vi "FRIC_navX_Get_Quaternion.vi"(6 "Zero":bool, 7 "Update":bool) -> (2 "Quaternion":T1)   [LabVIEW 2015, in "navX AE v1.lvlib"]
doc: "This navX VI returns the quaternion of the navX."
uses:
  navX AE v1.lvlib
  navX Library v2/_TypeDefs/Z900_navX_DeviceRegisters.ctl
  navX Library v2/navX Library v2.lvlib
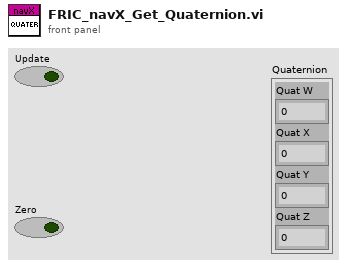
[diagram p1: front panel]
types:
  T1 = cluster{"Quat W":dbl, "Quat X":dbl, "Quat Y":dbl, "Quat Z":dbl}
  T2 = typedef "navX Library v2.lvlib/Z900_navX_DeviceRegisters.ctl" = u8
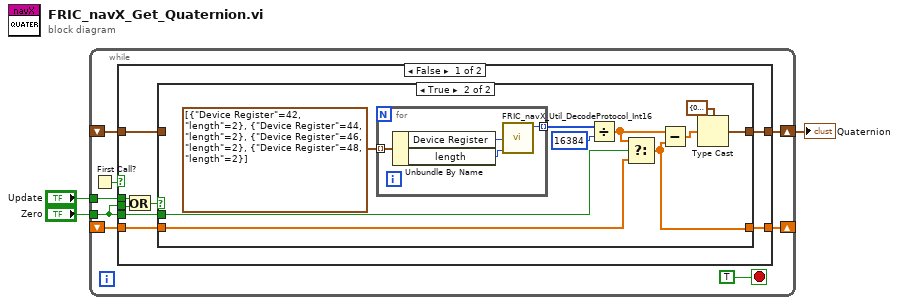
[diagram p0: block diagram]
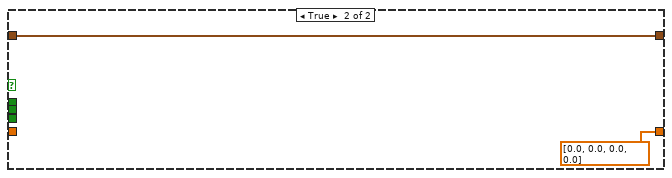
[diagram p3: hidden frame]
diagram:
  n1 = while {
    shift-right: [w11] -> w3
    shift-left: _ -> [w10]
    tunnel: "Update" -> [w8]
    tunnel: "Zero" -> [w5]
    shift-right: [w4] -> _
    shift-left: _ -> [w6]
    stop <- TRUE stop-if-true
    n2 = First Call?() -> (First Call?: T/F=w7:bool)
    n3 = case shown="False" w7 {
      tunnel: [w19 w37] -> w11
      tunnel: w10 -> [w18 w37]
      tunnel: w8 -> [w17 _]
      tunnel: w5 -> [w16 _]
      tunnel: w6 -> [w14 _]
      tunnel: w5 -> [w13 _]
      tunnel: [w12 dbl[] [0.0, 0.0, 0.0, 0.0]] -> w4
      frame False {
        n4 = Or(x=w17, y=w16) -> (x .or. y?=w15:bool)
        n5 = case shown="True" w15 {
          tunnel: [w21 w31] -> w19
          tunnel: w18 -> [w21 _]
          tunnel: w14 -> [w20 w24]
          tunnel: w13 -> [_ w23]
          tunnel: [w20 w22] -> w12
          frame False {
          }
          frame True {
            n6 = for {
              tunnel: cluster{"Device Register":T2, "length":i32}[] [{"Device Register"=42, "length"=2}, {"Device Register"=44, "length"=2}, {"Device Register"=46, "length"=2}, {"Device Register"=48, "length"=2}] ("Array") -> [w33] mode=indexing
              tunnel: [w32] -> w27 mode=indexing
              n7 = Unbundle By Name(w33) -> ("Device Register"=w35:T2, "length"=w34:i32)
              n8 = call "FRIC_navX_Util_DecodeProtocol_Int16.vi"("length"=w34, "Device Register"=w35) -> ("Value"=w32:i16)  [unwired: 9 in]
            }
            n9 = Divide(x=w27, y=u16 16384) -> (x/y=w25:dbl[])
            n10 = Select(t=w25, s=w23, f=w24) -> (s? t:f=w22:dbl[])
            n11 = Subtract(x=w25, y=w22) -> (x-y=w26:dbl[])
            n12 = Type Cast(type=T1 {"Quat W"=0.0, "Quat X"=0.0, "Quat Y"=0.0, "Quat Z"=0.0}, x=w26) -> (*(type *) &x=w31:T1)
          }
        }
      }
      frame True {
      }
    }
  }
  "Quaternion" <- w3
